vi "Lidar Test Global.vi"() -> ()   [LabVIEW 2010]
panel:
  out "ReadBit":bool
  in  "Write Bitarray":bool[](array[boolean])=[FALSE, FALSE, FALSE, FALSE, FALSE, FALSE, FALSE, FALSE]
  in  "Write Counter Outer":u16
  in  "Bitarray":bool[](array[boolean])=[FALSE, FALSE, FALSE, FALSE, FALSE, FALSE, FALSE, FALSE]
  out "Transmission Error":bool
  in  "Other Inner Loop Counter":u8
  out "Went Through":bool
  in  "Transmit Counter":u16
  in  "Read Counter Inner":u16
  in  "Read Counter Outer":u16
  in  "Test Val":u16
  in  "Magnitude":u16
  in  "Angle":u8
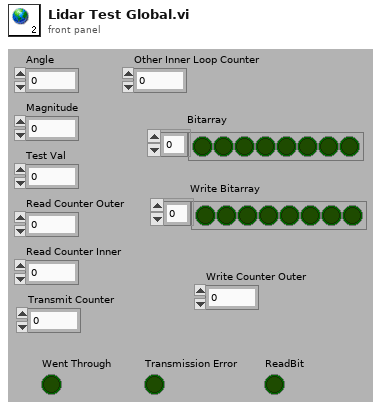
[diagram p1: front panel]
diagram:
